vi "Change Execution.vi"() -> ()   [LabVIEW 2016, in "xy_utilities.lvlib"]
uses:
  xy_utilities.lvlib
panel:
  out "Array":path[](array[path])
  out "Path":path
  in  "Edit Mode":bool
  in  "path":path
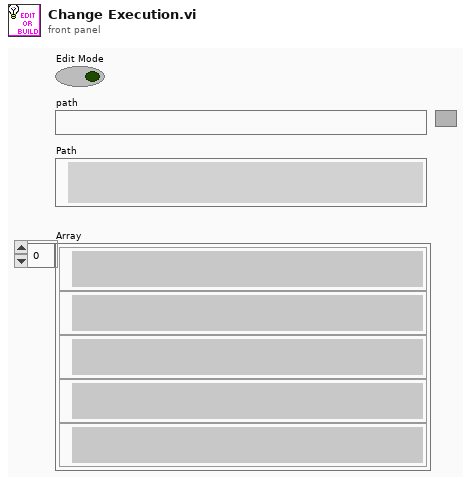
[diagram p1: front panel]
types:
  T1 = enum16{"Share clones between instances", "Preallocate clone for each instance"}
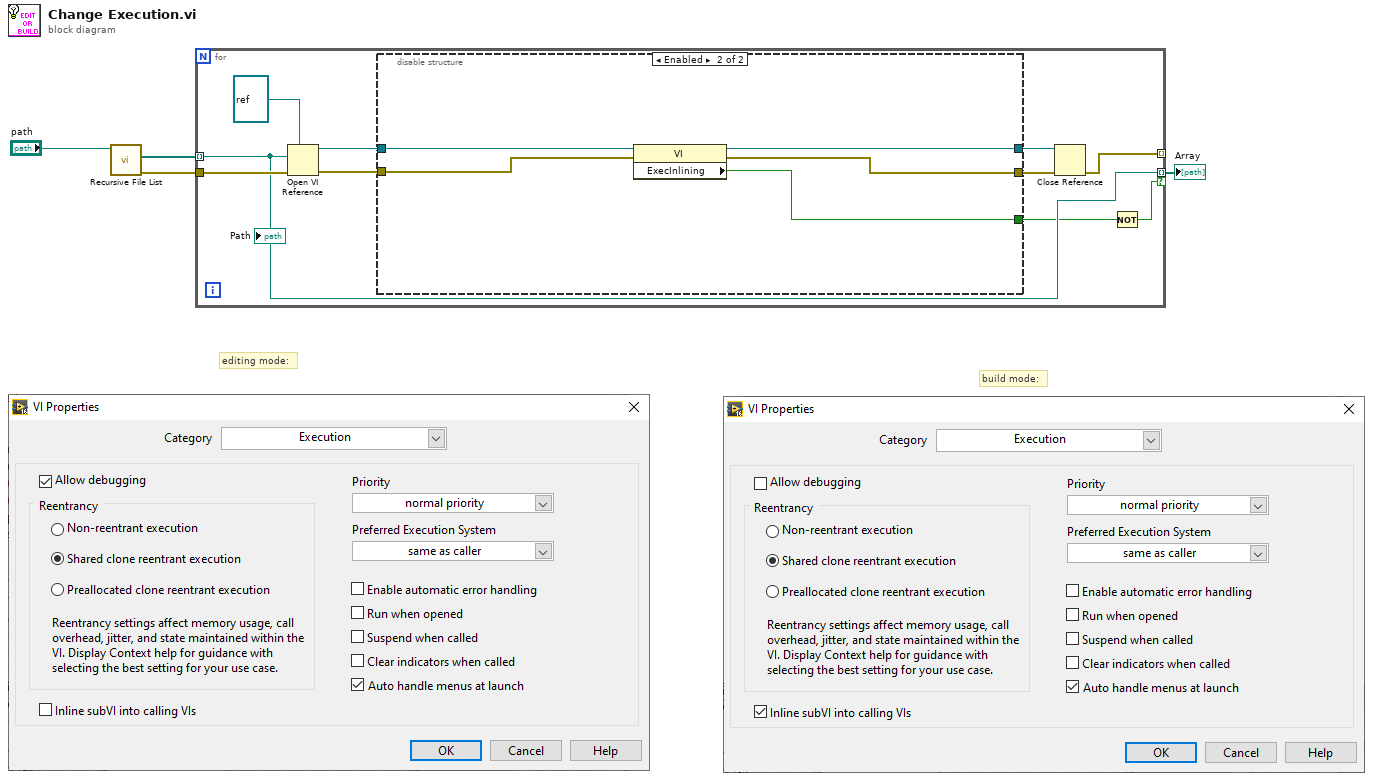
[diagram p0: block diagram]
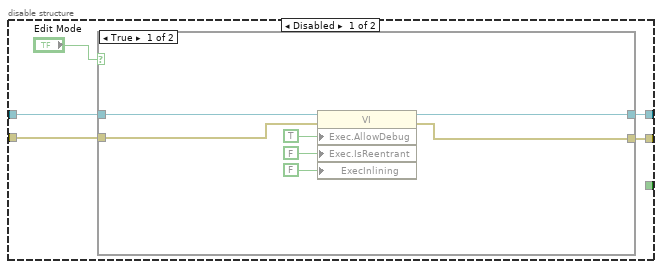
[diagram p2: hidden frame]
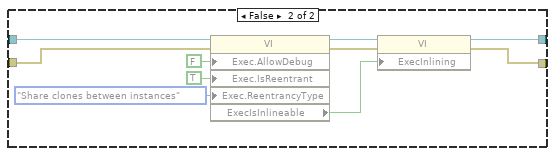
[diagram p3: hidden frame]
diagram:
  # "build mode:"
  # "editing mode:"
  n1 = call <vilib>:"Recursive File List.vi"("Folder Path"="path") -> ("error out"=w3:errorcluster, "All Files in Dir"=w2:path[])  [unwired: 6 in, 3 out]
  n2 = for {
    tunnel: w3 -> [w10]
    tunnel: w2 -> [w8] mode=indexing
    tunnel: [w8] -> w1 mode=indexing if=w5
    tunnel: [w7] -> _ mode=indexing
    n3 = Open VI Reference(type specifier VI Refnum (for type only)=refnum<vi> refnum, vi path=w8, error in (no error)=w10) -> (vi reference=w14:refnum<vi>, error out=w9:errorcluster)  [unwired: 3 in]
    n4 = disable-structure shown="Enabled" {
      disable-tunnel: w14 -> [w19 w41]
      disable-tunnel: [w18 w38] -> w12
      disable-tunnel: [w17 w39] -> w11
      disable-tunnel: w9 -> [w16 w40]
      disable-tunnel: [_ w37] -> w6
      frame Disabled {
        n5 = case shown="True" "Edit Mode" {
          tunnel: w19 -> [w26 w36]
          tunnel: [w25 w28] -> w18
          tunnel: [w24 w29] -> w17
          tunnel: w16 -> [w21 w33]
          frame True {
            n6 = property class="VI"(reference=w26, error in=w21, "Exec.AllowDebug"=TRUE ("Execution:Allow Debugging"), "Exec.IsReentrant"=FALSE ("Execution:Is Reentrant"), "ExecInlining"=FALSE ("Execution:Inline SubVI")) -> (reference out=w25:refnum<vi>, error out=w24:errorcluster)
          }
          frame False {
            n7 = property class="VI"(reference=w36, error in=w33, "Exec.AllowDebug"=FALSE ("Execution:Allow Debugging"), "Exec.IsReentrant"=TRUE ("Execution:Is Reentrant"), "Exec.ReentrancyType"=T1."Share clones between instances" ("Execution:Reentrancy Type")) -> (reference out=w31:refnum<vi>, error out=w30:errorcluster, "ExecIsInlineable"=w27:bool)
            n8 = property class="VI"(reference=w31, error in=w30, "ExecInlining"=w27) -> (reference out=w28:refnum<vi>, error out=w29:errorcluster)
          }
        }
      }
      frame Enabled {
        n9 = property class="VI"(reference=w41, error in=w40) -> (reference out=w38:refnum<vi>, error out=w39:errorcluster, "ExecInlining"=w37:bool)
      }
    }
    n10 = Close Reference(reference=w12, error in (no error)=w11) -> (error out=w7:errorcluster)
    n11 = Not(x=w6) -> (.not. x?=w5:bool)
    "Path" <- w8
  }
  "Array" <- w1
